vi "UI Refresh Data.vi"(8 "error in (no error)":errorcluster, 11 "GObject View in":refnum<class "RTM View.lvclass">) -> (0 "error out":errorcluster, 3 "GObject View out":refnum<class "RTM View.lvclass">)   [LabVIEW 2013, in "SET Project Editor.lvlib" / "RTM View.lvclass"]
uses:
  RTM View.lvclass
  UI View/UI View.lvclass/UI View.ctl
  RTM View.lvclass/RTM View.ctl
  SET Project Data/Project Data Class/Project Data.lvclass
  SET Project Data/Menu Class/Menu Data.lvclass/Menu Data.ctl
  UI View/Read _LangData.vi
  UI View/Read UUID.vi
  SET Project Data/Menu Class/Read Menu Path (Relative).vi
  SET Project Data/Menu Class/Read Menu Item LUT.vi
  SET Project Data/Menu Class/Read Languages.vi
  SET Project Editor.lvlib
  SET Project Data/Menu Class/Menu Data.lvclass
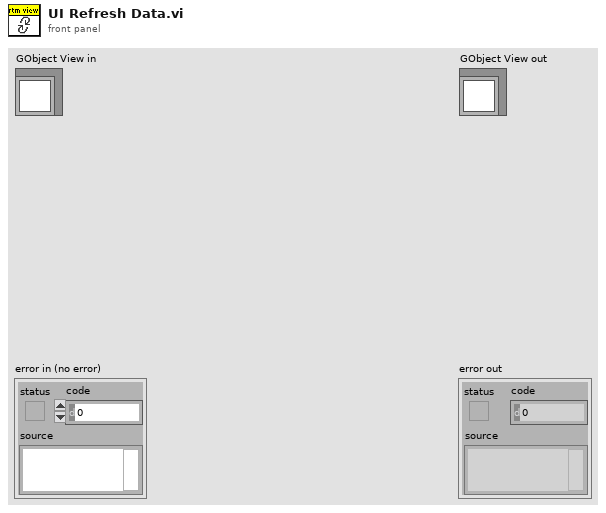
[diagram p1: front panel]
types:
  T1 = typedef "SET Resource File.lvlib/ResFile Lang Entry.ctl" = cluster{"Tag":string, "Name":string, "Code Page":u16}
  T2 = typedef "SET Project Data.lvlib/ProjFile_Resource Entry.ctl" = cluster{"RID":string, "Tag":string, "Strings [] (UTF-16)":string[], "Shared?":bool}
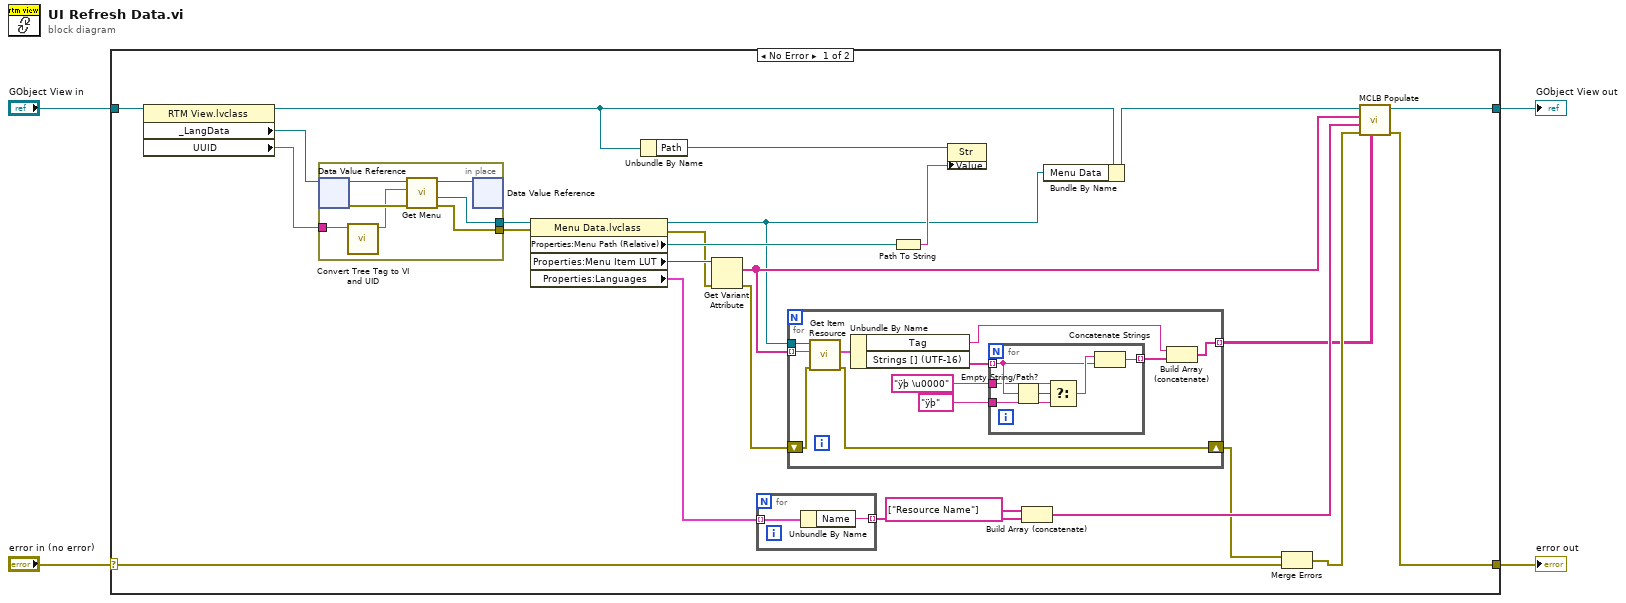
[diagram p0: block diagram]
diagram:
  n1 = case shown="No Error" "error in (no error)" {
    selector: "error in (no error)" -> [w23 w57]
    tunnel: [w20 w57] -> w3
    tunnel: [w19 w56] -> w1
    tunnel: "GObject View in" -> [w29 w56]
    frame No Error {
      n2 = property class="RTM View.lvclass"(reference=w29) -> (reference out=w16:refnum<class "RTM View.lvclass">, "_LangData"=w28:refnum<data-value>, "UUID"=w27:string)  [unwired: 1 in, 1 out]
      n3 = in-place {
        in-place-border: [w49] -> w8
        in-place-border: w27 -> [w52]
        in-place-border: [w50] -> w22
        n4 = in-place-dvr #1(w28) -> (w55:refnum<class "Project Data.lvclass">, w53:errorcluster)
        n5 = call "Convert Tree Tag to VI and UID.vi"("Tree Tag"=w52) -> ("File Path (Relative)"=w51:string)  [unwired: 7 in, 3 out]
        n6 = call-dynamic "Get Menu.vi"("error in (no error)"=w53, "Menu Path (Relative)"=w51, "ProjectData in"=w55) -> ("error out"=w49:errorcluster, "Menu Data out"=w50:refnum<class "Menu Data.lvclass">, "ProjectData out"=w54:refnum<class "Project Data.lvclass">)  [unwired: 5 in, 1 out]
        n7 = in-place-dvr #1(w54) -> ()  [unwired: 2 out]
      }
      n8 = property class="Menu Data.lvclass"(reference=w22, error in=w8) -> (reference out=w5:refnum<class "Menu Data.lvclass">, error out=w10:errorcluster, "Properties:Menu Path (Relative)"=w15:path, "Properties:Menu Item LUT"=w13:variant, "Properties:Languages"=w12:T1[])
      n9 = Unbundle By Name(w16) -> ("Path"=w26:refnum<vi>)
      n10 = Get Variant Attribute(Variant=w13, error in=w10) -> (names=w11:string[], error out=w9:errorcluster)  [unwired: 2 in, 2 out]
      n11 = for {
        tunnel: w12 -> [w48] mode=indexing
        tunnel: [w47] -> w17 mode=indexing
        n12 = Unbundle By Name(w48) -> ("Name"=w47:string)
      }
      n13 = for {
        shift-right: [w36] -> w7
        shift-left: w9 -> [w34]
        tunnel: [w37] -> w6 mode=indexing
        tunnel: w11 -> [w31] mode=indexing
        tunnel: w5 -> [w30]
        n14 = call "Get Item Resource.vi"("error in (no error)"=w34, "ItemName"=w31, "Menu Data in"=w30) -> ("error out"=w36:errorcluster, "Resource"=w35:T2)  [unwired: 4 in, 3 out]
        n15 = Unbundle By Name(w35) -> ("Tag"=w38:string, "Strings [] (UTF-16)"=w40:string[])
        n16 = for {
          tunnel: w40 -> [w44] mode=indexing
          tunnel: [w43] -> w39 mode=indexing
          tunnel: "ÿþ \u0000" ("string") -> [w42]
          tunnel: "ÿþ" ("string") -> [w41]
          n17 = Empty String/Path?(string/path=w44) -> (empty?=w46:bool)
          n18 = Select(t=w42, s=w46, f=w41) -> (s? t:f=w45:string)
          n19 = Concatenate Strings(w45, w44) -> (w43:string)
        }
        n20 = Build Array (concatenate)(w38, w39) -> (w37:string[])
      }
      n21 = Path To String(path=w15) -> (string=w14:string)
      n22 = property class="Str"(reference=w26, "Value"=w14) -> ()  [unwired: 1 in, 2 out]
      n23 = Build Array (concatenate)(string[] ["Resource Name"], w17) -> (w24:string[])
      n24 = Bundle By Name(cluster=w16, "Menu Data"=w5) -> (w18:refnum<class "RTM View.lvclass">)
      n25 = Merge Errors(w7, w23) -> (w21:errorcluster)
      n26 = call-dynamic "MCLB Populate.vi"("Item Names[][]"=w6, "error in (no error)"=w21, "Column Header Strings[]"=w24, "Row Header Strings[]"=w11, "View in"=w18) -> ("error out"=w20:errorcluster, "View out"=w19:refnum<class "RTM View.lvclass">)  [unwired: 5 in]
    }
    frame Error {
    }
  }
  "error out" <- w3
  "GObject View out" <- w1
